vi "convert_Time_JD_To_UTC0.vi"(8 "ut_Sec":dbl, 9 "Julian Date":dbl, 11 "UTC":dbl) -> (0 "UTC+0":dbl, 3 "Julian Date":dbl)   [LabVIEW 2015]
uses:
  <vilib>/imath/engines/lvmath2/RunTimeEngine/BuiltInFunctions/mod/NIMS_mod_no_size_check.vi
  <instcachedir>/0/NIMS_mod_no_size_check_5393E3382FD241D281EEB71DA286C65B.lvgen/NIMS_mod_no_size_check_5393E3382FD241D281EEB71DA286C65B_001.vi
  <vilib>/imath/engines/lvmath2/RunTimeEngine/NodeEndStatement/NIMS_NodeEndStatement_Output.vi
  <instcachedir>/0/NIMS_NodeEndStatement_Output_53EC0D466D134D7ABD903AC30B43404B.lvgen/NIMS_NodeEndStatement_Output_53EC0D466D134D7ABD903AC30B43404B_001.vi
  <vilib>/imath/engines/lvmath2/RunTimeEngine/ErrorHandling/NIMS_Finalize Error.vi
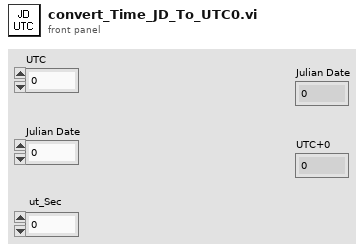
[diagram p1: front panel]
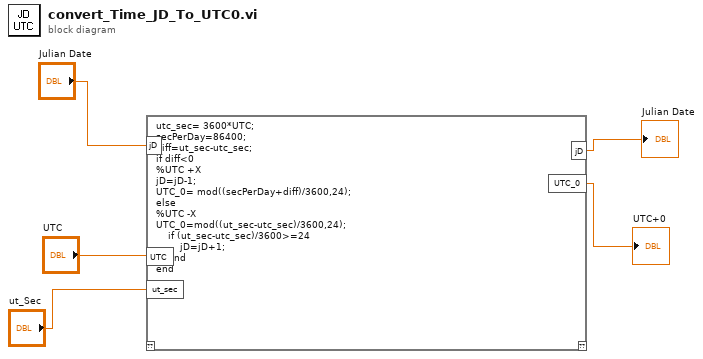
[diagram p0: block diagram]
diagram:
  n1 = mathscript code="utc_sec= 3600*UTC;\nsecPerDay=86400;\ndiff=ut_sec-utc_sec;\nif diff<0\n%UTC +X\njD=jD-1;\nUTC_0= mod((secPerDay+diff)/3600,24);\nelse\n%UTC -X\nUTC_0=mod((ut_sec-utc_sec)/3600,24);\n    if (ut_sec-utc_sec)/3600>=24\n        jD=jD+1;\n    end\nend" ("Nœud MathScript")("jD"="Julian Date", "UTC"="UTC", "ut_sec"="ut_Sec") -> ("UTC_0"=→"UTC+0":dbl, "jD"=→"Julian Date":dbl)  [unwired: 1 in, 1 out]
